vi "TCU Module (Main).vi"(7 "Name of Parent Panel":string="Main.vi", 9 "New Center Coords":T1={"Horizontal"=470, "Vertical"=200}, 10 "Config":variant, 11 "Main UI Message Queue":refnum<queue>) -> ()   [LabVIEW 2018, in "TCU Module.lvlib"]
doc: "This Continuous Measurement sample project is based on the Queued Message Handler template.\n\nThe Event Handling Loop generates messages based on user interface actions.\n\nThe Message Handling Loop processes messages generated by the Event Handling Loop, or by other messages. There are also Acquisition and Logging message handling loop subVIs, and a chart updating loop."
uses:
  TCU Module.lvlib
  support/Message Queue/Message Cluster.ctl
  <vilib>/Utility/miscctls.llb/LVPoint32TypeDef.ctl
  controls/UI Data.ctl
  controls/UI State.ctl
  TCU Module State Cluster.ctl
  TCU Module Config Cluster.ctl
  TCU Module Settings Cluster.ctl
  Measure Instrument/Output Devices.ctl
  Huber TCU/Huber Settings.ctl
  Lauda Integral XT-150 TCU/Lauda Settings.ctl
  Julabo Type 1 TCU/Julabo Type 1 TCU Folder/Julabo FP-50 Settings.ctl
  Huber Unistat 410 TCU/Huber Unistat 410 RS485 Settings.ctl
  Measure Instrument/State Enum.ctl
  TCU Module Display.ctl
  Sequencing/Squence Update Cluster.ctl
  support/Message Queue/Enqueue Message (Single).vi
  support/User Event - Stop/User Event - Stop.lvlib
  support/Support Library.lvlib
  support/Message Queue/Message Queue.lvlib
  Measure Instrument/TCU Module Engine.lvlib
  Measure Instrument/Feed Module Engine.lvlib
  Huber TCU/Huber Ministat 230 TCU.lvlib
  Lauda Integral XT-150 TCU/Lauda TCU.lvlib
  Julabo Type 1 TCU/Julabo Type 1 TCU Folder/Julabo Type FP-50 TCU.lvlib
  Sequencing/Sequencing Library.lvlib
  support/Command Log VIs/Command Logging.lvlib
  Huber Unistat 410 TCU/Huber Unistat 410 TCU.lvlib
panel:
  out "TCU On?":bool
  in  "Settings Button":bool
  out "TCU Image":u16(ring)
  out "ScanCode":i16
  out "Temp Display":dbl
  out "Log File path":path
  out "Status":string
  in  "Exit":bool
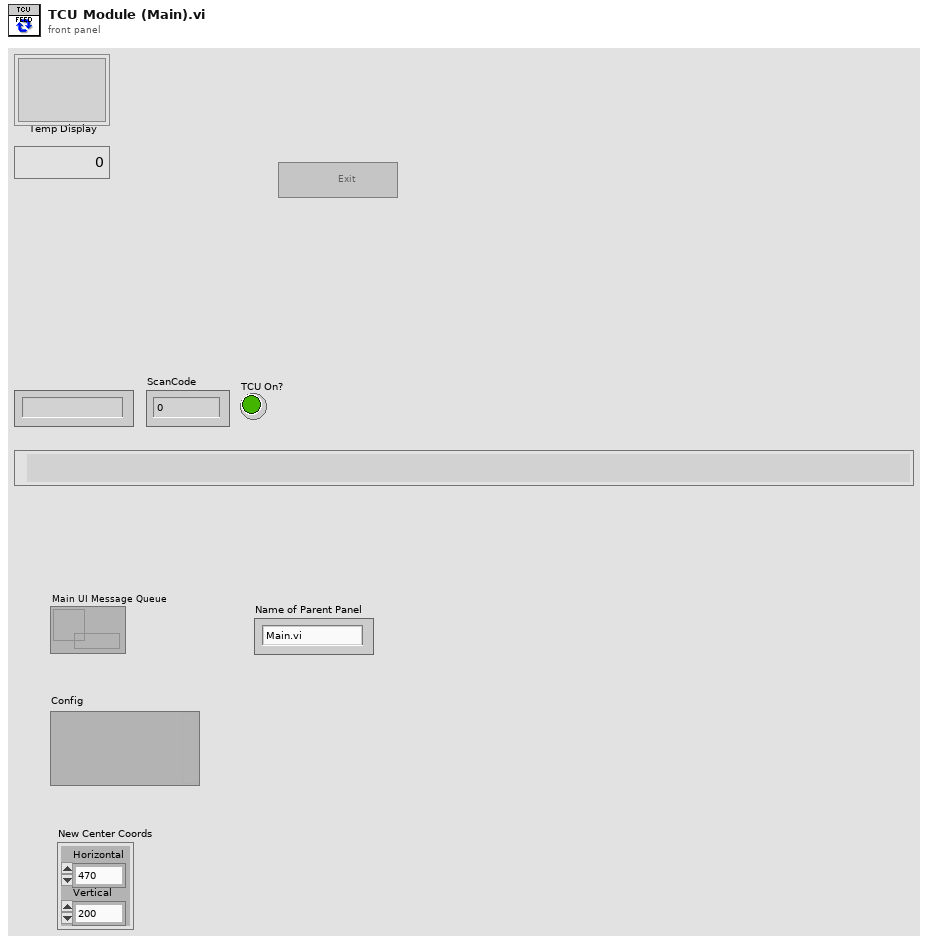
[diagram p1: front panel]
types:
  T1 = typedef "LVPoint32TypeDef.ctl" = cluster{"Horizontal":i32, "Vertical":i32}
  T2 = typedef "TCU Module.lvlib/TCU Module Config Cluster.ctl" = cluster{"GUID":string, "Drop Coords":T1, "Process Name":string, "Queue Name":string, "Settings":T3, "Load Count":i32, "Power Level Changed":bool}
  T3 = typedef "TCU Module.lvlib/TCU Module Settings Cluster.ctl" = cluster{"Cycle Period":dbl, "Setpoint Entry":dbl, "Output Device":T4, "Huber Ministat 230 Settings":T5, "Lauda Settings":T6, "Julabo FP-50 Settings":T7, "Internal Control?":bool, "Huber Unistat 410 Settings":T8}
  T4 = typedef "Output Devices.ctl" = enum16{"Default", "Huber Ministat 230", "Huber Unistat 410", "Lauda XT-150", "Julabo FP-50"}
  T5 = typedef "Huber Ministat 230 TCU.lvlib/Huber Settings.ctl" = cluster{"VISA resource name":refnum<visa-resource-name>, "Simulated?":bool}
  T6 = typedef "Lauda TCU.lvlib/Lauda Settings.ctl" = cluster{"VISA resource name":refnum<visa-resource-name>, "Simulated?":bool, "Pump Power":i32}
  T7 = typedef "Julabo Type FP-50 TCU.lvlib/Julabo FP-50 Settings.ctl" = cluster{"VISA resource name":refnum<visa-resource-name>, "Simulated?":bool, "Pump Power":i32}
  T8 = typedef "Huber Unistat 410 TCU.lvlib/Huber Unistat 410 RS485 Settings.ctl" = cluster{"VISA resource name":refnum<visa-resource-name>, "Address":i8, "Simulated?":bool}
  T9 = typedef "TCU Module.lvlib/TCU Module State Cluster.ctl" = cluster{"TCU Module Config":T2, "State":T10, "Start Time":timestamp, "Current Time":timestamp, "First Iteration":bool, "Data":cluster{"TCU Temp":dbl}, "Process Name":string, "TCU On?":bool, "Power Level Changed":bool}
  T10 = typedef "Feed Module.lvlib/Feed Module Engine.lvlib/State Enum.ctl" = enum16{"Measuring", "Idle", "Paused"}
  T11 = typedef "UI State.ctl" = enum16{"Idle", "Acquiring and Logging", "Waiting for Exit", "Waiting for Exit (Acq Stopped)", "Waiting for Exit (Log Stopped)", "Waiting for Stop", "Waiting for Stop (Acq Stopped)", "Waiting for Stop (Log Stopped)"}
  T12 = typedef "UI Data.ctl" = cluster{"Start Ref":refnum<vi>, "Trigger Ref":refnum<vi>, "Stop Ref":refnum<vi>, "Settings Ref":refnum<vi>, "Status Ref":refnum<vi>, "Exit Ref":refnum<vi>, "Data Ref":refnum<vi>}
  T13 = typedef "TCU Module.lvlib/All Message Queues.ctl" = cluster{"Engine":refnum<queue>, "TCU UI":refnum<queue>, "TCU Engine":refnum<queue>, "TCU Display":refnum<queue>}
  T14 = typedef "TCU Module.lvlib/TCU Module Display.ctl" = cluster{"TCU On?":bool, "Cycle Period":dbl, "Current TCU Temp":dbl}
  T15 = cluster{"Shift":bool, "Ctrl":bool, "Alt":bool, "Cmd":bool, "Opt":bool}
  T16 = typedef "Sequencing Library.lvlib/Squence Update Cluster.ctl" = cluster{"Auto?":bool, "Manual Entry":dbl, "Setpoint":dbl}
  T17 = enum8{"Enabled", "Disabled", "Disabled and Grayed Out"}
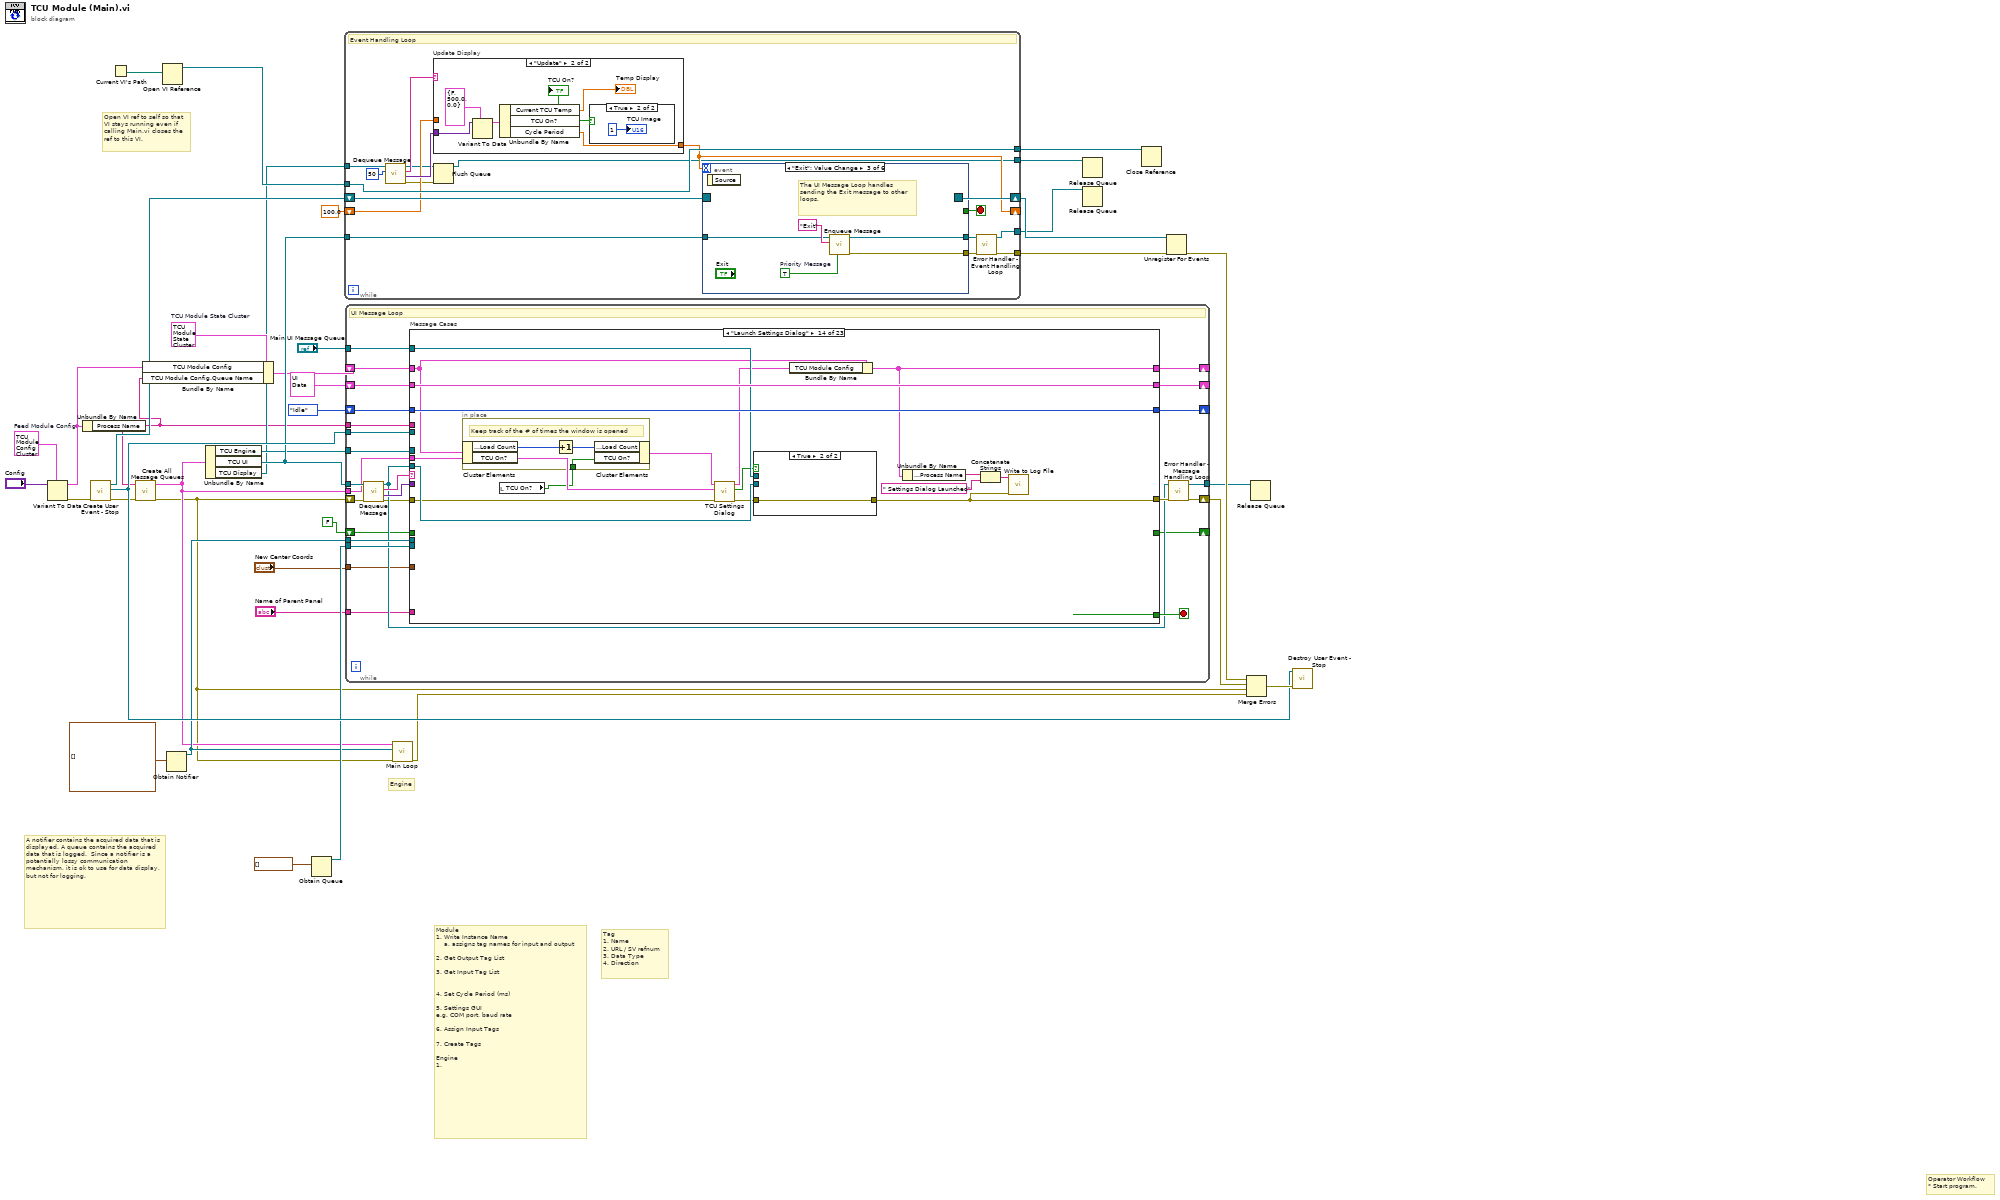
[diagram p0: block diagram]
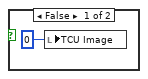
[diagram p3: hidden frame]
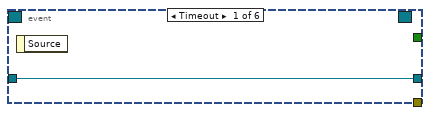
[diagram p4: hidden frame]
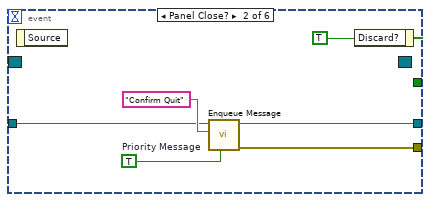
[diagram p5: hidden frame]
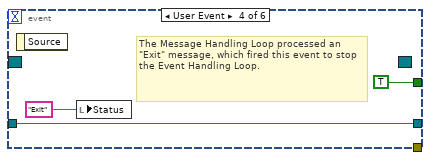
[diagram p6: hidden frame]
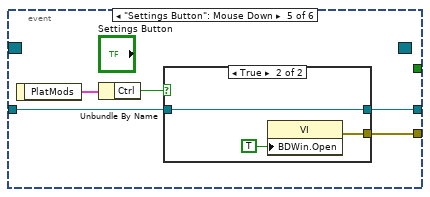
[diagram p7: hidden frame]
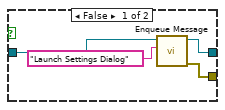
[diagram p8: hidden frame]
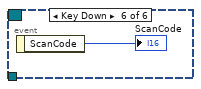
[diagram p9: hidden frame]
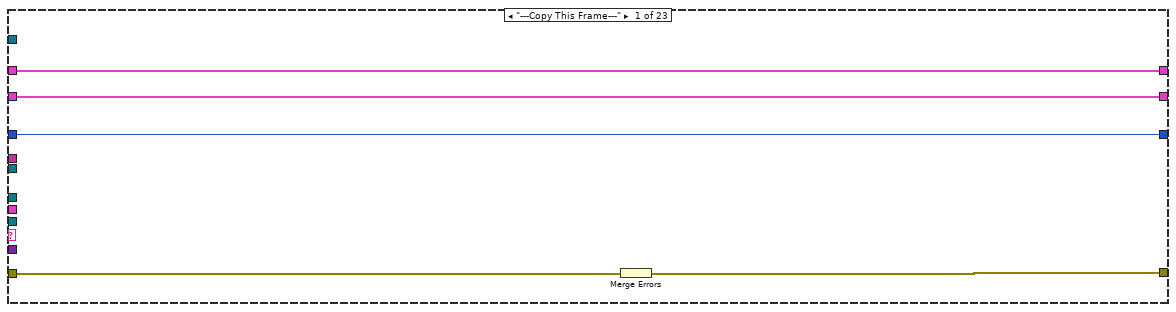
[diagram p10: hidden frame]
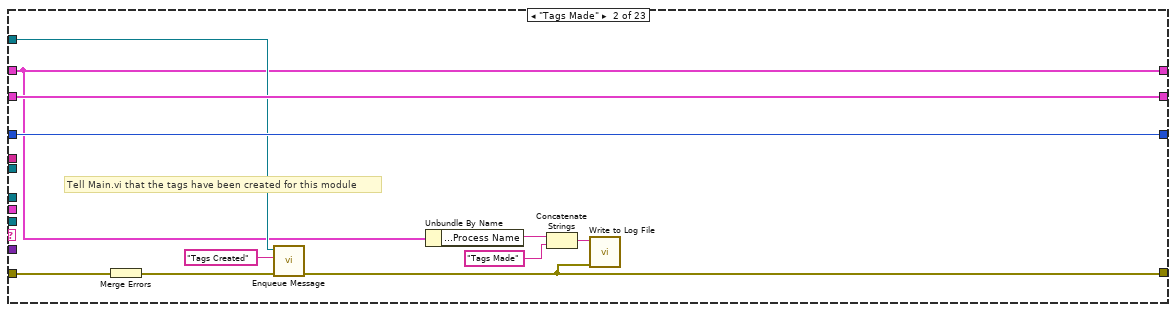
[diagram p11: hidden frame]
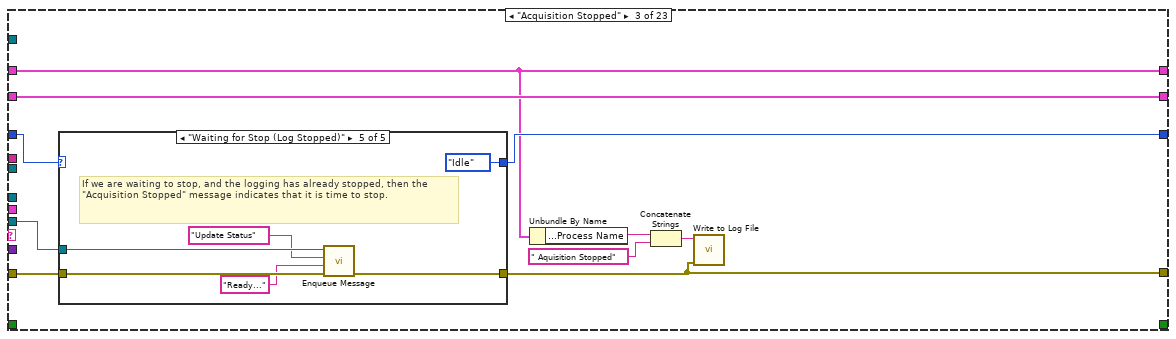
[diagram p12: hidden frame]
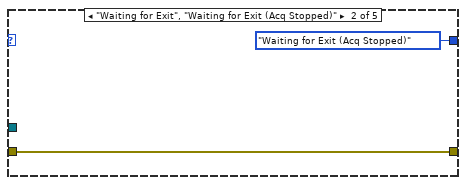
[diagram p14: hidden frame]
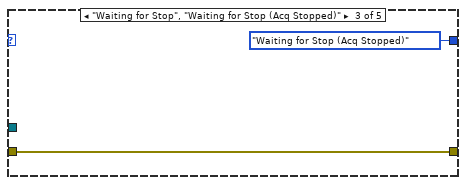
[diagram p15: hidden frame]
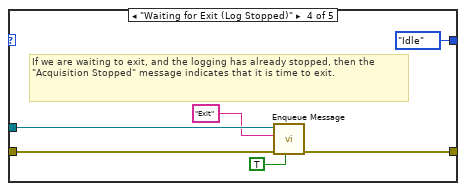
[diagram p16: hidden frame]
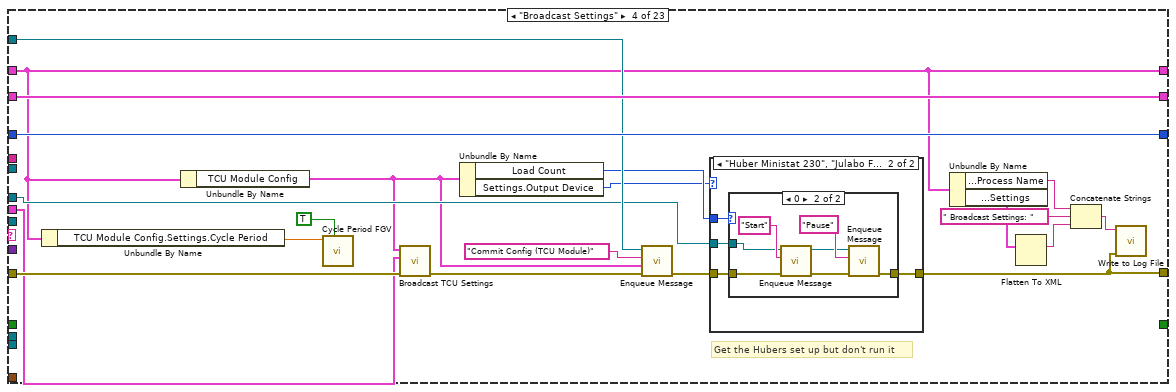
[diagram p17: hidden frame]
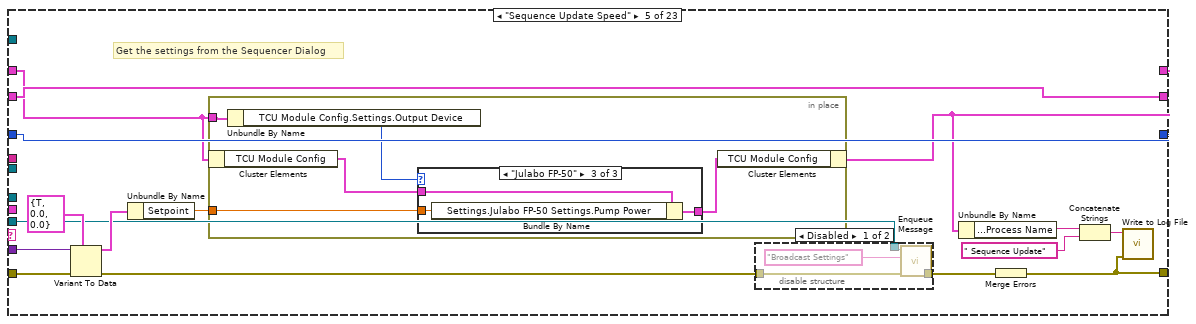
[diagram p20: hidden frame]
diagram:
  w12 = T2 {"GUID"="", "Drop Coords"={"Horizontal"=0, "Vertical"=0}, "Process Name"="", "Queue Name"="", "Settings"={"Cycle Period"=500.0, "Setpoint Entry"=0.0, "Output Device"=enum."Default", "Huber Ministat 230 Settings"={"VISA resource name"="", "Simulated?"=TRUE}, "Lauda Settings"={"VISA resource name"="", "Simulated?"=FALSE, "Pump Power"=2}, "Julabo FP-50 Settings"={"VISA resource name"="", "Simulated?"=FALSE, "Pump Power"=2}, "Internal Control?"=FALSE, "Huber Unistat 410 Settings"={"VISA resource name"="", "Address"=0, "Simulated?"=FALSE}}, "Load Count"=0, "Power Level Changed"=FALSE}  # Feed Module Config
  w15 = T9 {"TCU Module Config"={"GUID"="", "Drop Coords"={"Horizontal"=0, "Vertical"=0}, "Process Name"="", "Queue Name"="", "Settings"={"Cycle Period"=500.0, "Setpoint Entry"=0.0, "Output Device"=enum."Default", "Huber Ministat 230 Settings"={"VISA resource name"="", "Simulated?"=TRUE}, "Lauda Settings"={"VISA resource name"="", "Simulated?"=FALSE, "Pump Power"=2}, "Julabo FP-50 Settings"={"VISA resource name"="", "Simulated?"=FALSE, "Pump Power"=2}, "Internal Control?"=FALSE, "Huber Unistat 410 Settings"={"VISA resource name"="", "Address"=0, "Simulated?"=FALSE}}, "Load Count"=0, "Power Level Changed"=FALSE}, "State"=enum."Idle", "Start Time"=timestamp(0 s since 1904-01-01), "Current Time"=timestamp(0 s since 1904-01-01), "First Iteration"=FALSE, "Data"={"TCU Temp"=0.0}, "Process Name"="", "TCU On?"=FALSE, "Power Level Changed"=FALSE}  # TCU Module State Cluster
  # "Open VI ref to self so that\nVI stays running even if\ncalling Main.vi closes the\nref to this VI."
  # "Engine"
  # "Operator Workflow\n* Start program."
  # "Module \n1. Write Instance Name\n    a. assigns tag names for input and output\n\n2. Get Output Tag List\n\n3. Get Input Tag List\n\n\n4. Set Cycle Period (ms)\n\n5. Settings GUI\ne.g. COM port, baud rate\n\n6. Assign Input Tags\n\n7. Create Tags\n\nEngine\n1."
  # "Tag\n1. Name\n2. URL / SV refnum\n3. Data Type\n4. Direction"
  # "A notifier contains the acquired data that is displayed. A queue contains the acquired data that is logged.  Since a notifier is a potentially lossy communication mechanism, it is ok to use for data display, but not for logging."
  n1 = Variant To Data(type=w12, Variant="Config") -> (data=w17:T2, error out=w18:errorcluster)  [unwired: 1 in]
  n2 = Unbundle By Name(w17) -> ("Process Name"=w5:string)
  n3 = call "Create User Event - Stop.vi"("error in (no error)"=w18) -> ("error out"=w11:errorcluster, "User Event - Stop"=w34:refnum<user-event>, "Stop Event Registration Refnum"=w35:refnum<event-registration>)  [unwired: 8 in]
  n4 = Current VI's Path() -> (path=w20:path)
  n5 = call "Create All Message Queues.vi"("error in (no error)"=w11, "Process Name"=w5) -> ("error out"=w9:errorcluster, "Message Queues"=w10:T13)  [unwired: 8 in]
  n6 = Bundle By Name(cluster=w15, "TCU Module Config"=w17, "TCU Module Config.Queue Name"=w5) -> (w19:T9)
  n7 = Open VI Reference(vi path=w20) -> (vi reference=w21:refnum<vi>)  [unwired: 5 in, 1 out]
  n8 = Obtain Notifier(notification data type=waveform(dbl)[] []) -> (notifier out=w23:refnum<notifier>)  [unwired: 3 in, 2 out]
  n9 = Unbundle By Name(w10) -> ("TCU Engine"=w26:refnum<queue>, "TCU UI"=w30:refnum<queue>, "TCU Display"=w14:refnum<queue>)
  n10 = Obtain Queue(element data type=waveform(dbl)[] []) -> (queue out=w25:refnum<queue>)  [unwired: 4 in, 2 out]
  n11 = while {
    tunnel: w30 -> [w50]
    tunnel: [w52] -> w37
    shift-right: [w51] -> w32
    shift-left: w35 -> [w56]
    tunnel: [w49] -> w22
    tunnel: w21 -> [w49]
    tunnel: w14 -> [w48]
    shift-right: [w45] -> _
    shift-left: 100.0 ("Cycle Period") -> [w44]
    tunnel: [w40] -> w2
    tunnel: [w39] -> w3
    stop <- w55 stop-if-true
    # "Event Handling Loop"
    n12 = call "Dequeue Message.vi"("timeout in ms (-1)"=50, "Message Queue"=w48) -> ("error out"=w41:errorcluster, "Message Data"=w46:variant, "Message"=w47:string, "dup Message Queue"=w42:refnum<queue>)  [unwired: 6 in]
    n13 = case "Update Display" shown="\"Update\"" w47 {
      tunnel: w46 -> [_ w63]
      tunnel: [w57 w59] -> w45
      tunnel: w44 -> [w57 _]
      frame "False", Default {
      }
      frame "Update" {
        n14 = Variant To Data(type=T14 {"TCU On?"=FALSE, "Cycle Period"=500.0, "Current TCU Temp"=0.0} ("FM Display"), Variant=w63) -> (data=w62:T14)  [unwired: 1 in, 1 out]
        n15 = Unbundle By Name(w62) -> ("Current TCU Temp"=→"Temp Display":dbl, "TCU On?"=w60:bool, "Cycle Period"=w59:dbl)
        "TCU On?" <- w60
        n16 = case shown="True" w60 {
          frame False {
            n17 = local write "TCU Image"(u16 0 ("Ring")) -> ()
          }
          frame True {
            "TCU Image" <- u16 1 ("Ring")
          }
        }
      }
    }
    n18 = Flush Queue(queue=w42, error in (no error)=w41) -> (queue out=w39:refnum<queue>)  [unwired: 2 out]
    n19 = event shown="[2] \"Exit\": Value Change" {
      selector: w56 -> [_ _ _ _ _ _]
      dyn-events: [_ _ _ _ _ _] -> w51
      timeout: w45 -> [_ _ _ _ _ _]
      tunnel: [_ _ _ TRUE ("Discard?") _ _] -> w55
      tunnel: w50 -> [w66 w69 w74 w78 w83 _]
      tunnel: [_ w67 w77 _ w85 _] -> w53
      tunnel: [w66 w68 w73 w78 w84 _] -> w54
      event Timeout {
        n20 = event-data() -> ()  [unwired: 1 in, 1 out]
      }
      event Panel Close? {
        w70 = TRUE  # Priority Message
        n21 = event-data() -> ()  [unwired: 1 in, 1 out]
        n22 = call-poly "Enqueue Message.vi"("Priority Message? (F)"=w70, "Message"="Confirm Quit", "Message Queue"=w69) -> ("error out"=w67:errorcluster, "dup Message Queue"=w68:refnum<queue>)  [unwired: 7 in]
        n23 = event-data("Discard?"=TRUE) -> ()  [unwired: 1 in, 1 out]
      }
      event "Exit": Value Change {
        w75 = TRUE  # Priority Message
        # "The UI Message Loop handles sending the Exit message to other loops."
        n24 = event-data() -> ()  [unwired: 1 in, 1 out]
        n25 = call-poly "Enqueue Message.vi"("Priority Message? (F)"=w75, "Message"="Exit", "Message Queue"=w74) -> ("error out"=w77:errorcluster, "dup Message Queue"=w73:refnum<queue>)  [unwired: 7 in]
      }
      event User Event {
        # "The Message Handling Loop processed an \"Exit\" message, which fired this event to stop the Event Handling Loop."
        n26 = event-data() -> ()  [unwired: 1 in, 1 out]
        n27 = local write "Status"("Exit" ("Exit String")) -> ()
      }
      event "Settings Button": Mouse Down {
        n28 = event-data() -> ("PlatMods"=w82:T15)  [unwired: 1 in]
        n29 = Unbundle By Name(w82) -> ("Ctrl"=w81:bool)
        n30 = case shown="True" w81 {
          tunnel: [w89 w90] -> w85
          tunnel: [w88 w91] -> w84
          tunnel: w83 -> [w87 w91]
          frame False {
            n31 = call-poly "Enqueue Message.vi"("Message"="Launch Settings Dialog", "Message Queue"=w87) -> ("error out"=w89:errorcluster, "dup Message Queue"=w88:refnum<queue>)  [unwired: 8 in]
          }
          frame True {
            n32 = property class="VI"("BDWin.Open"=TRUE ("Block Diagram Window:Open")) -> (error out=w90:errorcluster)  [unwired: 2 in, 1 out]
          }
        }
      }
      event Key Down {
        n33 = event-data() -> ("ScanCode"=→"ScanCode":i16)  [unwired: 1 in]
      }
    }
    n34 = call "Error Handler - Event Handling Loop.vi"("error in (no error)"=w53, "Message Queue"=w54) -> ("dup error in"=w52:errorcluster, "dup Message Queue"=w40:refnum<queue>)  [unwired: 8 in]
  }
  n35 = while {
    tunnel: w30 -> [w115]
    tunnel: w34 -> [w119]
    shift-right: [w109] -> w38
    shift-left: w9 -> [w118]
    shift-right: [w101] -> _
    shift-left: w19 -> [w103]
    shift-right: [w113] -> _
    shift-left: T12 {"Start Ref"=refnum, "Trigger Ref"=refnum, "Stop Ref"=refnum, "Settings Ref"=refnum, "Status Ref"=refnum, "Exit Ref"=refnum, "Data Ref"=refnum} ("Measurement UI Controls") -> [w114]
    tunnel: w23 -> [w112]
    tunnel: w25 -> [w111]
    shift-right: [w106] -> _
    shift-left: UI_State."Idle" ("UI State") -> [w107]
    tunnel: w26 -> [w105]
    tunnel: "Main UI Message Queue" -> [w102]
    tunnel: w10 -> [w100]
    tunnel: w5 -> [w99]
    tunnel: "New Center Coords" -> [w98]
    tunnel: "Name of Parent Panel" -> [w97]
    shift-right: [w96] -> _
    shift-left: FALSE -> [w95]
    tunnel: [w94] -> w1
    stop <- w120 stop-if-true
    # "UI Message Loop"
    n36 = call "Dequeue Message.vi"("error in (no error)"=w118, "Message Queue"=w115) -> ("error out"=w104:errorcluster, "Message Data"=w116:variant, "Message"=w117:string, "dup Message Queue"=w108:refnum<queue>)  [unwired: 6 in]
    n37 = case "Message Cases" shown="\"Launch Settings Dialog\"" w117 {
      selector: w117 -> [_ _ _ _ _ _ _ _ _ _ _ _ _ _ _ _ _ _ _ _ _ _ w620]
      tunnel: w108 -> [_ _ w142 _ w207 w239 w258 _ w325 w339 w364 _ w402 w422 w443 _ w489 w520 _ _ w573 _ _]
      tunnel: w104 -> [w125 w136 w143 w181 w206 w238 w257 w293 w306 w343 w368 w387 w397 w420 w444 w469 w487 w519 w539 w553 w571 w612 _]
      tunnel: [w124 w126 w139 w168 w201 w233 w255 w294 w300 w330 w346 w387 w389 w413 w439 w473 w478 w505 w547 w555 w576 w613 w619] -> w110
      tunnel: [_ _ _ _ _ _ _ _ _ _ TRUE _ _ _ _ _ _ _ _ _ _ _ _] -> w120
      tunnel: w116 -> [_ _ _ _ w205 w237 _ w296 _ w342 w350 _ _ _ _ w466 _ _ _ _ _ w611 _]
      tunnel: w119 -> [_ _ _ _ _ _ _ _ _ _ w367 _ _ _ _ _ _ _ _ _ _ _ _]
      tunnel: w103 -> [w121 w127 w138 w167 w200 w232 w254 w291 w304 w329 w345 w378 w388 w410 w438 w471 w483 w515 w540 w554 w581 w602 w625]
      tunnel: w114 -> [w123 w135 w146 w185 w209 w241 w260 w298 w322 w344 w365 w386 w398 w425 w447 w476 w484 w516 w546 w564 w597 w608 w630]
      tunnel: [w123 w135 w146 w185 w209 w241 w260 w298 w322 w344 w365 w385 w398 w425 w447 w476 w484 w516 w546 w564 w597 w608 w630] -> w113
      tunnel: w112 -> [_ _ _ _ _ _ _ _ _ _ w363 _ _ _ _ _ _ _ _ _ _ _ _]
      tunnel: w111 -> [_ _ _ _ _ _ _ _ _ _ w359 _ _ _ _ _ _ _ _ _ _ _ _]
      tunnel: w107 -> [w122 w134 w145 w184 w208 w240 w259 w292 w311 w334 _ _ _ w424 w446 w472 _ _ _ _ w586 w603 w629]
      tunnel: [w122 w134 w144 w184 w208 w240 w256 w292 w312 w334 UI_State."Idle" ("UI State") UI_State."Idle" ("UI State") UI_State."Idle" ("UI State") w424 w445 w472 UI_State."Acquiring and Logging" ("UI State") UI_State."Acquiring and Logging" ("UI State") UI_State."Acquiring and Logging" ("UI State") UI_State."Acquiring and Logging" ("UI State") w587 w603 w629] -> w106
      tunnel: w105 -> [_ _ _ w174 _ _ _ _ w310 _ w357 _ _ _ _ _ _ _ w544 w562 w585 _ _]
      tunnel: w102 -> [_ w132 _ w180 _ _ _ _ _ _ w351 _ _ w423 _ _ _ _ _ _ _ _ _]
      tunnel: [w121 w127 w138 w167 w199 w231 w254 w291 w299 w329 w345 w378 w388 w412 w438 w471 w477 w504 w540 w554 w575 w602 w625] -> w101
      tunnel: w100 -> [_ _ _ w177 _ _ _ _ _ _ _ _ _ w417 _ _ _ _ _ _ _ _ _]
      tunnel: w99 -> [_ _ _ _ _ _ _ _ _ _ _ _ w393 _ _ _ _ _ _ _ _ _ _]
      tunnel: w98 -> [_ _ _ _ _ _ _ _ _ _ _ _ w395 _ _ _ _ _ _ _ _ _ _]
      tunnel: w97 -> [_ _ _ _ _ _ _ _ _ _ _ _ w394 _ _ _ _ _ _ _ _ _ _]
      tunnel: w95 -> [_ _ _ _ _ _ _ _ _ _ _ _ _ _ _ _ _ w510 _ _ _ _ _]
      tunnel: [_ _ _ _ _ _ _ _ _ _ _ _ _ _ _ _ _ w509 _ _ _ _ _] -> w96
      frame "---Copy This Frame---" {
        # "Duplicate this frame when creating new messages.  Change this comment in the duplicated frame to describe this message."
        n38 = Merge Errors(w125) -> (w124:errorcluster)
      }
      frame "Tags Made" {
        # "Tell Main.vi that the tags have been created for this module"
        # "Duplicate this frame when creating new messages.  Change this comment in the duplicated frame to describe this message."
        n39 = Merge Errors(w136) -> (w131:errorcluster)
        n40 = call-poly "Enqueue Message.vi"("error in (no error)"=w131, "Message"="Tags Created", "Message Queue"=w132) -> ("error out"=w126:errorcluster)  [unwired: 7 in, 1 out]
        n41 = Unbundle By Name(w127) -> ("TCU Module Config.Process Name"=w130:string)
        n42 = Concatenate Strings(w130, "Tags Made" ("text")) -> (w128:string)
        n43 = call "Write to Log File.vi"("error in"=w126, "text"=w128) -> ()  [unwired: 9 in, 1 out]
      }
      frame "Acquisition Stopped" {
        # "Logic for determining what action to take when the acquisition has stopped."
        n44 = case shown="\"Waiting for Stop (Log Stopped)\"" w145 {
          selector: w145 -> [w148 _ _ _ _]
          tunnel: [w148 UI_State."Waiting for Exit (Acq Stopped)" ("UI State") UI_State."Waiting for Stop (Acq Stopped)" ("UI State") UI_State."Idle" ("UI State") UI_State."Idle" ("UI State")] -> w144
          tunnel: w143 -> [w147 w149 w151 w157 w163]
          tunnel: [w147 w149 w151 w156 w162] -> w139
          tunnel: w142 -> [_ _ _ w155 w161]
          frame Default {
          }
          frame "Waiting for Exit", "Waiting for Exit (Acq Stopped)" {
          }
          frame "Waiting for Stop", "Waiting for Stop (Acq Stopped)" {
          }
          frame "Waiting for Exit (Log Stopped)" {
            # "If we are waiting to exit, and the logging has already stopped, then the \"Acquisition Stopped\" message indicates that it is time to exit."
            n45 = call-poly "Enqueue Message.vi"("Priority Message? (F)"=TRUE, "error in (no error)"=w157, "Message"="Exit", "Message Queue"=w155) -> ("error out"=w156:errorcluster)  [unwired: 6 in, 1 out]
          }
          frame "Waiting for Stop (Log Stopped)" {
            # "If we are waiting to stop, and the logging has already stopped, then the \"Acquisition Stopped\" message indicates that it is time to stop."
            n46 = call-poly "Enqueue Message.vi"("error in (no error)"=w163, "Message Data"="Ready..." ("Message"), "Message"="Update Status", "Message Queue"=w161) -> ("error out"=w162:errorcluster)  [unwired: 6 in, 1 out]
          }
        }
        n47 = Unbundle By Name(w138) -> ("TCU Module Config.Process Name"=w141:string)
        n48 = Concatenate Strings(w141, " Aquisition Stopped" ("text")) -> (w140:string)
        n49 = call "Write to Log File.vi"("error in"=w139, "text"=w140) -> ()  [unwired: 9 in, 1 out]
      }
      frame "Broadcast Settings" {
        # "Get the Hubers set up but don't run it"
        # "Send the 'Update Settings' message to the Logging and Acquisition message loops."
        n50 = Unbundle By Name(w167) -> ("TCU Module Config.Settings.Cycle Period"=w182:dbl)
        n51 = Unbundle By Name(w167) -> ("TCU Module Config"=w172:T2)
        n52 = call "Cycle Period FGV.vi"("Write"=TRUE, "Cycle Period In (ms)"=w182) -> ()  [unwired: 8 in, 2 out]
        n53 = call "Broadcast TCU Settings.vi"("error in (no error)"=w181, "Message Queues"=w177, "Pump Module Config"=w172) -> ("error out"=w179:errorcluster)  [unwired: 8 in]
        n54 = Unbundle By Name(w172) -> ("Load Count"=w176:i32, "Settings.Output Device"=w173:T4)
        n55 = call-poly "Enqueue Message.vi"("error in (no error)"=w179, "Message Data"=w172, "Message"="Commit Config (TCU Module)", "Message Queue"=w180) -> ("error out"=w175:errorcluster)  [unwired: 6 in, 1 out]
        n56 = case shown="\"Huber Ministat 230\", \"Julabo FP-50\"" w173 {
          tunnel: w175 -> [w186 w190]
          tunnel: w174 -> [_ w189]
          tunnel: [w186 w188] -> w168
          tunnel: w176 -> [_ w187]
          frame "Default", Default {
          }
          frame "Huber Ministat 230", "Julabo FP-50" {
            n57 = case shown="0" w187 {
              tunnel: w190 -> [w191 w195]
              tunnel: w189 -> [_ w194]
              tunnel: [w191 w198] -> w188
              frame Default {
              }
              frame 0 {
                n58 = call-poly "Enqueue Message.vi"("error in (no error)"=w195, "Message"="Start", "Message Queue"=w194) -> ("error out"=w192:errorcluster, "dup Message Queue"=w193:refnum<queue>)  [unwired: 7 in]
                n59 = call-poly "Enqueue Message.vi"("error in (no error)"=w192, "Message"="Pause", "Message Queue"=w193) -> ("error out"=w198:errorcluster)  [unwired: 7 in, 1 out]
              }
            }
          }
        }
        n60 = Unbundle By Name(w167) -> ("TCU Module Config.Process Name"=w171:string, "TCU Module Config.Settings"=w166:T3)
        n61 = Flatten To XML(anything=w166) -> (xml string=w165:string)
        n62 = Concatenate Strings(w171, " Broadcast Settings: " ("text"), w165) -> (w170:string)
        n63 = call "Write to Log File.vi"("error in"=w168, "text"=w170) -> ()  [unwired: 9 in, 1 out]
      }
      frame "Sequence Update Speed" {
        # "Get the settings from the Sequencer Dialog"
        # "Send the 'Update Settings' message to the Logging and Acquisition message loops."
        n64 = Variant To Data(error in=w206, type=T16 {"Auto?"=TRUE, "Manual Entry"=0.0, "Setpoint"=0.0} ("Cluster"), Variant=w205) -> (data=w213:T16, error out=w210:errorcluster)
        n65 = Unbundle By Name(w213) -> ("Setpoint"=w212:dbl)
        n66 = in-place {
          in-place-border: w212 -> [w223]
          in-place-border: w200 -> [w222]
          n67 = in-place-cluster #1(w200) -> ("TCU Module Config"=w220:T2)
          n68 = Unbundle By Name(w222) -> ("TCU Module Config.Settings.Output Device"=w221:T4)
          n69 = case shown="\"Julabo FP-50\"" w221 {
            tunnel: w220 -> [w224 w227 w230]
            tunnel: w223 -> [_ w226 w229]
            tunnel: [w224 w225 w228] -> w219
            frame "Default", Default {
            }
            frame "Lauda XT-150" {
              n70 = Bundle By Name(cluster=w227, "Settings.Lauda Settings.Pump Power"=w226) -> (w225:T2)
            }
            frame "Julabo FP-50" {
              n71 = Bundle By Name(cluster=w230, "Settings.Julabo FP-50 Settings.Pump Power"=w229) -> (w228:T2)
            }
          }
          n72 = in-place-cluster #1("TCU Module Config"=w219) -> (w199:T9)
        }
        n73 = disable-structure shown="Disabled" {
          disable-tunnel: [w218 _] -> w211
          disable-tunnel: w210 -> [w216 _]
          disable-tunnel: w207 -> [w215 _]
          frame Disabled {
            n74 = call-poly "Enqueue Message.vi"("error in (no error)"=w216, "Message"="Broadcast Settings", "Message Queue"=w215) -> ("error out"=w218:errorcluster)  [unwired: 7 in, 1 out]
          }
          frame Enabled {
          }
        }
        n75 = Unbundle By Name(w199) -> ("TCU Module Config.Process Name"=w204:string)
        n76 = Merge Errors(w211) -> (w201:errorcluster)
        n77 = Concatenate Strings(w204, " Sequence Update" ("text")) -> (w203:string)
        n78 = call "Write to Log File.vi"("error in"=w201, "text"=w203) -> ()  [unwired: 9 in, 1 out]
      }
      frame "Sequence Update Temperature" {
        # "Get the settings from the Sequencer Dialog"
        # "Send the 'Update Settings' message to the Logging and Acquisition message loops."
        n79 = Variant To Data(error in=w238, type=T16 {"Auto?"=TRUE, "Manual Entry"=0.0, "Setpoint"=0.0} ("Cluster"), Variant=w237) -> (data=w245:T16, error out=w242:errorcluster)
        n80 = Unbundle By Name(w245) -> ("Setpoint"=w244:dbl)
        n81 = in-place {
          in-place-border: w244 -> [w253]
          n82 = in-place-cluster #2(w232) -> ("TCU Module Config"=w251:T2)
          n83 = Bundle By Name(cluster=w251, "Settings.Setpoint Entry"=w253) -> (w252:T2)
          n84 = in-place-cluster #2("TCU Module Config"=w252) -> (w231:T9)
        }
        n85 = disable-structure shown="Disabled" {
          disable-tunnel: [w250 _] -> w243
          disable-tunnel: w242 -> [w248 _]
          disable-tunnel: w239 -> [w247 _]
          frame Disabled {
            n86 = call-poly "Enqueue Message.vi"("error in (no error)"=w248, "Message"="Broadcast Settings", "Message Queue"=w247) -> ("error out"=w250:errorcluster)  [unwired: 7 in, 1 out]
          }
          frame Enabled {
          }
        }
        n87 = Unbundle By Name(w231) -> ("TCU Module Config.Process Name"=w236:string)
        n88 = Merge Errors(w243) -> (w233:errorcluster)
        n89 = Concatenate Strings(w236, " Sequence Update" ("text")) -> (w235:string)
        n90 = call "Write to Log File.vi"("error in"=w233, "text"=w235) -> ()  [unwired: 9 in, 1 out]
      }
      frame "Confirm Quit" {
        # "Confirm Quit - Message that can confirm whether or not the user wants to exit the application."
        n91 = case shown="\"Acquiring and Logging\"" w259 {
          tunnel: w258 -> [w269 w276]
          tunnel: w257 -> [w268 w274]
          tunnel: [w262 w273] -> w255
          tunnel: [UI_State."Idle" ("UI State") w272] -> w256
          tunnel: w254 -> [w261 w271]
          frame Default {
            # "If 'Confirm Quit' comes in while the system is idle, there is no need for a confirmation message."
            n92 = call-poly "Enqueue Message.vi"("Priority Message? (F)"=TRUE, "error in (no error)"=w268, "Message"="Exit", "Message Queue"=w269) -> ("error out"=w262:errorcluster)  [unwired: 6 in, 1 out]
            n93 = Unbundle By Name(w261) -> ("TCU Module Config.Process Name"=w265:string)
            n94 = Concatenate Strings(w265, " Quit" ("text")) -> (w264:string)
            n95 = call "Write to Log File.vi"("error in"=w262, "text"=w264) -> ()  [unwired: 9 in, 1 out]
          }
          frame "Acquiring and Logging" {
            n96 = Two Button Dialog(message="Are you sure you want to quit while the acquisition is running?" ("Confirm Quit Message"), 1:"No" ("No"), 2:"Yes" ("Yes")) -> (T button?=w275:bool)
            n97 = case shown="True" w275 {
              tunnel: w276 -> [_ w290]
              tunnel: w274 -> [w280 w289]
              tunnel: [w280 w283] -> w273
              tunnel: [UI_State."Acquiring and Logging" ("UI State") UI_State."Waiting for Exit" ("UI State")] -> w272
              tunnel: w271 -> [_ w282]
              frame False {
                # "User did not want to quit."
              }
              frame True {
                n98 = call-poly "Enqueue Message.vi"("error in (no error)"=w289, "Message"="Stop", "Message Queue"=w290) -> ("error out"=w283:errorcluster)  [unwired: 7 in, 1 out]
                n99 = Unbundle By Name(w282) -> ("TCU Module Config.Process Name"=w286:string)
                n100 = Concatenate Strings(w286, " Quit" ("text")) -> (w285:string)
                n101 = call "Write to Log File.vi"("error in"=w283, "text"=w285) -> ()  [unwired: 9 in, 1 out]
              }
            }
          }
        }
      }
      frame "Display Log File Path" {
        n102 = Variant To Data(error in=w293, type=path "", Variant=w296) -> (data=→"Log File path":path, error out=w294:errorcluster)
      }
      frame "E-Stop" {
        # "Pause the TCU when E-Stop is pressed"
        # "Message Acquisition and Logging loops to stop"
        # "Enable: Start, Exit, Settings\nDisable: Stop"
        # "Stop the pumps."
        n103 = Unbundle By Name(w322) -> ("Trigger Ref"=w313:refnum<vi>, "Stop Ref"=w314:refnum<vi>, "Start Ref"=w317:refnum<vi>, "Exit Ref"=w316:refnum<vi>, "Settings Ref"=w315:refnum<vi>)
        n104 = call-poly "Enqueue Message.vi"("error in (no error)"=w306, "Message Data"="Ready..." ("Ready..."), "Message"="Update Status", "Message Queue"=w325) -> ("error out"=w308:errorcluster)  [unwired: 6 in, 1 out]
        n105 = Build Array(w317, w316, w315) -> (w320:refnum<vi>[])
        n106 = Build Array(w313, w314) -> (w319:refnum<vi>[])
        n107 = call-poly "Enqueue Message.vi"("error in (no error)"=w308, "Message"="Pause", "Message Queue"=w310) -> ("error out"=w307:errorcluster)  [unwired: 7 in, 1 out]
        n108 = call "Set Enable State on Multiple Controls.vi"("Enable?"=FALSE, "Controls"=w319) -> ()  [unwired: 10 in]
        n109 = call "Set Enable State on Multiple Controls.vi"("Enable?"=TRUE, "Controls"=w320) -> ()  [unwired: 10 in]
        n110 = case shown="Default" w311 {
          selector: w311 -> [_ w327]
          tunnel: [UI_State."Waiting for Stop" ("UI State") w327] -> w312
          frame Default {
          }
          frame "Waiting for Exit" {
          }
        }
        n111 = Bundle By Name(cluster=w304, "State"=State_Enum."Idle") -> (w299:T9)
        n112 = Merge Errors(w307) -> (w300:errorcluster)
        n113 = Unbundle By Name(w299) -> ("TCU Module Config.Process Name"=w303:string)
        n114 = Concatenate Strings(w303, " E-STOP" ("text")) -> (w302:string)
        n115 = call "Write to Log File.vi"("error in"=w300, "text"=w302) -> ()  [unwired: 9 in, 1 out]
      }
      frame "Error" {
        # "Error - Check the error message data and respond accordingly. This message is sent by the \"Error Handler\" VIs at the end of each loop in this application."
        n116 = Variant To Data(error in=w343, type=errorcluster {"status"=FALSE, "code"=0, "source"=""} ("error out"), Variant=w342) -> (data=w340:errorcluster, error out=w336:errorcluster)
        n117 = call <vilib>:"General Error Handler.vi"("error in (no error)"=w340) -> ("message"=w328:string)  [unwired: 10 in, 4 out]
        n118 = call-poly "Enqueue Message.vi"("Priority Message? (F)"=TRUE, "Message"="Exit", "Message Queue"=w339) -> ("error out"=w335:errorcluster)  [unwired: 7 in, 1 out]
        n119 = Merge Errors(w335, w336) -> (w330:errorcluster)
        n120 = Unbundle By Name(w329) -> ("TCU Module Config.Process Name"=w333:string)
        n121 = Concatenate Strings(w333, " Error: " ("text"), w328) -> (w332:string)
        n122 = call "Write to Log File.vi"("error in"=w330, "text"=w332) -> ()  [unwired: 9 in, 1 out]
      }
      frame "Exit" {
        w354 = TRUE  # Delete Module?
        # "Don't check the error outs. The acquisition and logging queues may have already been released."
        # "Close references owned by the Main VI."
        # "Stop the VI"
        # "Exit - Fire the User Event to stop the Event Handling Loop.  Also send Exit messages to the Acquisition and Logging loops."
        n123 = Release Queue(queue=w364, error in (no error)=w368) -> (error out=w362:errorcluster)  [unwired: 1 in, 2 out]
        n124 = call "Fire User Event - Stop.vi"("User Event - Stop"=w367) -> ("error out"=w366:errorcluster)  [unwired: 10 in]
        n125 = Release Notifier(notifier=w363, error in (no error)=w362) -> (error out=w361:errorcluster)  [unwired: 1 in, 2 out]
        n126 = Build Array(w357) -> (w356:refnum<queue>[])
        n127 = Release Queue(queue=w359, error in (no error)=w361) -> (error out=w360:errorcluster)  [unwired: 1 in, 2 out]
        n128 = for {
          tunnel: w356 -> [w375] mode=indexing
          n129 = call-poly "Enqueue Message.vi"("Message"="Stop", "Message Queue"=w375) -> ("dup Message Queue"=w376:refnum<queue>)  [unwired: 8 in, 1 out]
          n130 = call-poly "Enqueue Message.vi"("Message"="Exit", "Message Queue"=w376) -> ()  [unwired: 8 in, 2 out]
        }
        n131 = Variant To Data(type=w354, Variant=w350) -> (data=w353:bool, error out=w355:errorcluster)  [unwired: 1 in]
        n132 = Select(t=w354, s=w355, f=w353) -> (s? t:f=w352:bool)
        n133 = case "Don't enqueue Delete Module if opening campaign because it\nwill already have been deleted and new config loaded and we create\na race condition." shown="True" w352 {
          tunnel: w351 -> [_ w372]
          tunnel: w345 -> [_ w371]
          frame False {
          }
          frame True {
            n134 = Unbundle By Name(w371) -> ("TCU Module Config.GUID"=w370:string)
            n135 = call-poly "Enqueue Message.vi"("Message Data"=w370, "Message"="Delete Module", "Message Queue"=w372) -> ()  [unwired: 7 in, 2 out]
          }
        }
        n136 = Merge Errors(w366, w360) -> (w346:errorcluster)
        n137 = Unbundle By Name(w345) -> ("TCU Module Config.Process Name"=w349:string)
        n138 = Concatenate Strings(w349, " Exit" ("text")) -> (w348:string)
        n139 = call "Write to Log File.vi"("error in"=w346, "text"=w348) -> ()  [unwired: 9 in, 1 out]
      }
      frame "Init UI Refs" {
        # "Enable: Start, Exit, Settings\nDisable: Stop"
        # "Init UI Refs - Store control references for UI controls.  Also enable/disable controls appropriately."
        n140 = property class="VI"("Front Panel.Closeable"=TRUE ("Front Panel Window:Closeable")) -> ()  [unwired: 2 in, 2 out]
        n141 = control-ref of="Status"() -> (w383:refnum<vi>)
        n142 = control-ref of="Exit"() -> (w380:refnum<vi>)
        n143 = Bundle By Name(cluster=w386, "Status Ref"=w383, "Exit Ref"=w380) -> (w385:T12)
        n144 = Build Array(w380) -> (w382:refnum<vi>[])
        n145 = call "Set Enable State on Multiple Controls.vi"("Enable?"=TRUE, "Controls"=w382) -> ()  [unwired: 10 in]
      }
      frame "Initialize" {
        # "Initialize - Get configuration settings, then message the UI to initialize, and broadcast the settings to the other message loops."
        n146 = property class="VI" props=["FP.State"]() -> (reference out=w396:refnum<vi>)  [unwired: 2 in, 2 out]
        n147 = call-poly "Enqueue Message.vi"("error in (no error)"=w397, "Message"="Init UI Refs", "Message Queue"=w402) -> ("error out"=w400:errorcluster, "dup Message Queue"=w401:refnum<queue>)  [unwired: 7 in]
        n148 = call "Make Child and Move.vi"("Process Name"=w393, "Name of Parent Panel"=w394, "New Center Coords"=w395, "VI in"=w396) -> ()  [unwired: 8 in]
        n149 = call-poly "Enqueue Message.vi"("error in (no error)"=w400, "Message"="Broadcast Settings", "Message Queue"=w401) -> ("error out"=w408:errorcluster, "dup Message Queue"=w407:refnum<queue>)  [unwired: 7 in]
        n150 = call-poly "Enqueue Message.vi"("error in (no error)"=w408, "Message Data"="Ready..." ("Ready..."), "Message"="Update Status", "Message Queue"=w407) -> ("error out"=w389:errorcluster)  [unwired: 6 in, 1 out]
        n151 = Unbundle By Name(w388) -> ("TCU Module Config.Process Name"=w392:string)
        n152 = Concatenate Strings(w392, " Initialize" ("text")) -> (w391:string)
        n153 = call "Write to Log File.vi"("error in"=w389, "text"=w391) -> ()  [unwired: 9 in, 1 out]
      }
      frame "Launch Settings Dialog" {
        # "Launch the Settings Dialog when the user clicks the 'Settings' button."
        n154 = local read "TCU On?"() -> (w411:bool)
        n155 = in-place {
          in-place-border: w411 -> [w426]
          # "Keep track of the # of times the window is opened"
          n156 = in-place-cluster #3(w410) -> ("TCU Module Config.Load Count"=w428:i32)  [unwired: 1 out]
          n157 = Increment(x=w428) -> (x+1=w427:i32)
          n158 = in-place-cluster #3("TCU Module Config.Load Count"=w427, "TCU On?"=w426) -> (w409:T9)
        }
        n159 = call "TCU Settings Dialog.vi"("error in (no error)"=w420, "Message Queues"=w417, "TCU Module State Cluster In"=w409) -> ("error out"=w419:errorcluster, "UI Refresh Needed?"=w418:bool, "TCU Module Config Out"=w421:T2)  [unwired: 5 in, 1 out]
        n160 = case shown="True" w418 {
          tunnel: w419 -> [w431 w437]
          tunnel: [w429 w437] -> w413
          tunnel: w423 -> [_ _]
          tunnel: w422 -> [w430 _]
          frame False {
            n161 = disable-structure shown="Enabled" {
              disable-tunnel: w431 -> [w435 w436]
              disable-tunnel: w430 -> [w434 _]
              disable-tunnel: [w432 w436] -> w429
              frame Disabled {
                n162 = call-poly "Enqueue Message.vi"("error in (no error)"=w435, "Message"="Broadcast Settings", "Message Queue"=w434) -> ("error out"=w432:errorcluster)  [unwired: 7 in, 1 out]
              }
              frame Enabled {
              }
            }
          }
          frame True {
          }
        }
        n163 = Bundle By Name(cluster=w410, "TCU Module Config"=w421) -> (w412:T9)
        n164 = Unbundle By Name(w412) -> ("TCU Module Config.Process Name"=w416:string)
        n165 = Concatenate Strings(w416, " Settings Dialog Launched" ("text")) -> (w415:string)
        n166 = call "Write to Log File.vi"("error in"=w413, "text"=w415) -> ()  [unwired: 9 in, 1 out]
      }
      frame "Logging Stopped" {
        # "Logic for determining what action to take when the logging has stopped."
        n167 = case shown="\"Waiting for Exit (Acq Stopped)\"" w446 {
          selector: w446 -> [w449 _ _ _ _]
          tunnel: [w449 UI_State."Waiting for Exit (Log Stopped)" ("UI State") UI_State."Waiting for Stop (Log Stopped)" ("UI State") UI_State."Idle" ("UI State") UI_State."Idle" ("UI State")] -> w445
          tunnel: w444 -> [w448 w450 w452 w458 w464]
          tunnel: [w448 w450 w452 w457 w463] -> w439
          tunnel: w443 -> [_ _ _ w456 w462]
          frame Default {
          }
          frame "Waiting for Exit", "Waiting for Exit (Log Stopped)" {
          }
          frame "Waiting for Stop", "Waiting for Stop (Log Stopped)" {
          }
          frame "Waiting for Exit (Acq Stopped)" {
            # "If we are waiting to exit, and the acquisition has already stopped, then the \"Logging Stopped\" message indicates that it is time to exit."
            n168 = call-poly "Enqueue Message.vi"("Priority Message? (F)"=TRUE, "error in (no error)"=w458, "Message"="Exit", "Message Queue"=w456) -> ("error out"=w457:errorcluster)  [unwired: 6 in, 1 out]
          }
          frame "Waiting for Stop (Acq Stopped)" {
            # "If we are waiting to stop, and the acquisition has already stopped, then the \"Logging Stopped\" message indicates that it is time to stop."
            n169 = call-poly "Enqueue Message.vi"("error in (no error)"=w464, "Message Data"="Ready..." ("Message"), "Message"="Update Status", "Message Queue"=w462) -> ("error out"=w463:errorcluster)  [unwired: 6 in, 1 out]
          }
        }
        n170 = Unbundle By Name(w438) -> ("TCU Module Config.Process Name"=w442:string)
        n171 = Concatenate Strings(w442, " Logging Stopped" ("text")) -> (w441:string)
        n172 = call "Write to Log File.vi"("error in"=w439, "text"=w441) -> ()  [unwired: 9 in, 1 out]
      }
      frame "Send to Sequence" {
        n173 = Variant To Data(error in=w469, type=refnum<queue> refnum ("Message Queue"), Variant=w466) -> (data=w467:refnum<queue>, error out=w468:errorcluster)
        n174 = local read "Temp Display"() -> (w474:dbl)
        n175 = call-poly "Enqueue Message.vi"("error in (no error)"=w468, "Message Data"=w474, "Message"="Sent to Sequence", "Message Queue"=w467) -> ("error out"=w473:errorcluster)  [unwired: 6 in, 1 out]
      }
      frame "Start" {
        # "Clear chart"
        # "Message Acquisition and Logging loops to start"
        # "Enable: Stop\nDisable: Start, Exit, Settings"
        # "Start - Enable/Disable buttons appropriately for an acquisition that has started, and update status display."
        n176 = Unbundle By Name(w484) -> ("Trigger Ref"=w495:refnum<vi>, "Stop Ref"=w496:refnum<vi>, "Start Ref"=w499:refnum<vi>, "Exit Ref"=w498:refnum<vi>, "Settings Ref"=w497:refnum<vi>, "Data Ref"=w486:refnum<vi>)
        n177 = property class="WFChart (strict)"(reference=w486, "History Data"=waveform(dbl)[][] []) -> ()  [unwired: 1 in, 2 out]
        n178 = Build Array(w499, w498, w497) -> (w502:refnum<vi>[])
        n179 = Build Array(w495, w496) -> (w501:refnum<vi>[])
        n180 = call-poly "Enqueue Message.vi"("error in (no error)"=w487, "Message"="Broadcast settings", "Message Queue"=w489) -> ("error out"=w490:errorcluster, "dup Message Queue"=w488:refnum<queue>)  [unwired: 7 in]
        n181 = call "Set Enable State on Multiple Controls.vi"("Enable?"=TRUE, "Controls"=w501) -> ()  [unwired: 10 in]
        n182 = call "Set Enable State on Multiple Controls.vi"("Enable?"=FALSE, "Controls"=w502) -> ()  [unwired: 10 in]
        n183 = call-poly "Enqueue Message.vi"("error in (no error)"=w490, "Message"="Start Loops", "Message Queue"=w488) -> ("error out"=w491:errorcluster)  [unwired: 7 in, 1 out]
        n184 = Merge Errors(w491) -> (w478:errorcluster)
        n185 = Bundle By Name(cluster=w483, "State"=State_Enum."Measuring") -> (w477:T9)
        n186 = Unbundle By Name(w477) -> ("TCU Module Config.Process Name"=w481:string)
        n187 = Concatenate Strings(w481, " Start" ("text")) -> (w480:string)
        n188 = call "Write to Log File.vi"("error in"=w478, "text"=w480) -> ()  [unwired: 9 in, 1 out]
      }
      frame "Sequence Start" {
        # "Start the sequence if it is not already running"
        # "Clear chart"
        # "Message Acquisition and Logging loops to start"
        # "Enable: Stop\nDisable: Start, Exit, Settings"
        # "Start - Enable/Disable buttons appropriately for an acquisition that has started, and update status display."
        n189 = Unbundle By Name(w516) -> ("Trigger Ref"=w523:refnum<vi>, "Stop Ref"=w524:refnum<vi>, "Start Ref"=w527:refnum<vi>, "Exit Ref"=w526:refnum<vi>, "Settings Ref"=w525:refnum<vi>, "Data Ref"=w518:refnum<vi>)
        n190 = property class="WFChart (strict)"(reference=w518, "History Data"=waveform(dbl)[][] []) -> ()  [unwired: 1 in, 2 out]
        n191 = Build Array(w527, w526, w525) -> (w530:refnum<vi>[])
        n192 = Build Array(w523, w524) -> (w529:refnum<vi>[])
        n193 = call-poly "Enqueue Message.vi"("error in (no error)"=w519, "Message"="Broadcast settings", "Message Queue"=w520) -> ("error out"=w512:errorcluster, "dup Message Queue"=w513:refnum<queue>)  [unwired: 7 in]
        n194 = call "Set Enable State on Multiple Controls.vi"("Enable?"=TRUE, "Controls"=w529) -> ()  [unwired: 10 in]
        n195 = call "Set Enable State on Multiple Controls.vi"("Enable?"=FALSE, "Controls"=w530) -> ()  [unwired: 10 in]
        n196 = case shown="False" w510 {
          selector: w510 -> [_ w537]
          tunnel: [TRUE w537] -> w509
          tunnel: w512 -> [w535 w538]
          tunnel: w513 -> [w533 _]
          tunnel: [w532 w538] -> w511
          frame False {
            n197 = call-poly "Enqueue Message.vi"("error in (no error)"=w535, "Message"="Start Loops", "Message Queue"=w533) -> ("error out"=w532:errorcluster)  [unwired: 7 in, 1 out]
          }
          frame True {
          }
        }
        n198 = Merge Errors(w511) -> (w505:errorcluster)
        n199 = Bundle By Name(cluster=w515, "State"=State_Enum."Measuring") -> (w504:T9)
        n200 = Unbundle By Name(w504) -> ("TCU Module Config.Process Name"=w508:string)
        n201 = Concatenate Strings(w508, " Sequence Start" ("text")) -> (w507:string)
        n202 = call "Write to Log File.vi"("error in"=w505, "text"=w507) -> ()  [unwired: 9 in, 1 out]
      }
      frame "Start Loops" {
        # "We don't have multiple Process Names per module, but i am leaving it for now."
        # "Message Acquisition and Logging loops to start"
        # "Start - Enable/Disable buttons appropriately for an acquisition that has started, and update status display."
        n203 = Unbundle By Name(w540) -> ("TCU Module Config.Process Name"=w541:string)
        n204 = Build Array(w544) -> (w542:refnum<queue>[])
        n205 = for {
          tunnel: w539 -> [w551]
          tunnel: [w550] -> w543 mode=indexing
          tunnel: w542 -> [w549] mode=indexing
          tunnel: w541 -> [w548]
          n206 = call-poly "Enqueue Message.vi"("error in (no error)"=w551, "Message Data"=w548, "Message"="Start", "Message Queue"=w549) -> ("error out"=w550:errorcluster)  [unwired: 6 in, 1 out]
        }
        n207 = property class="VI"("Front Panel.Title"=w541) -> ()  [unwired: 2 in, 2 out]
        n208 = Merge Errors(w539, w543) -> (w547:errorcluster)
      }
      frame "Start Log" {
        # "Message Acquisition and Logging loops to start"
        # "Start - Enable/Disable buttons appropriately for an acquisition that has started, and update status display."
        n209 = Unbundle By Name(w554) -> ("TCU Module Config.Process Name"=w559:string)
        n210 = Build Array(w562) -> (w560:refnum<queue>[])
        n211 = for {
          tunnel: w553 -> [w568]
          tunnel: [w567] -> w561 mode=indexing
          tunnel: w560 -> [w566] mode=indexing
          tunnel: w559 -> [w565]
          n212 = call-poly "Enqueue Message.vi"("error in (no error)"=w568, "Message Data"=w565, "Message"="Start Log", "Message Queue"=w566) -> ("error out"=w567:errorcluster)  [unwired: 6 in, 1 out]
        }
        n213 = property class="VI"("Front Panel.Title"=w559) -> ()  [unwired: 2 in, 2 out]
        n214 = Merge Errors(w553, w561) -> (w555:errorcluster)
        n215 = Unbundle By Name(w554) -> ("TCU Module Config.Process Name"=w558:string)
        n216 = Concatenate Strings(w558, " Start Log" ("text")) -> (w557:string)
        n217 = call "Write to Log File.vi"("error in"=w555, "text"=w557) -> ()  [unwired: 9 in, 1 out]
      }
      frame "Stop" {
        # "Pause the TCU on Stop"
        # "Enable: Start, Exit, Settings\nDisable: Stop"
        # "Stop - Enable/Disable buttons appropriately for an acquisition that has stopped, and update status display."
        n218 = Unbundle By Name(w597) -> ("Trigger Ref"=w588:refnum<vi>, "Stop Ref"=w589:refnum<vi>, "Start Ref"=w592:refnum<vi>, "Exit Ref"=w591:refnum<vi>, "Settings Ref"=w590:refnum<vi>)
        n219 = call-poly "Enqueue Message.vi"("error in (no error)"=w571, "Message"="Broadcast settings", "Message Queue"=w573) -> ("error out"=w570:errorcluster, "dup Message Queue"=w572:refnum<queue>)  [unwired: 7 in]
        n220 = Build Array(w592, w591, w590) -> (w595:refnum<vi>[])
        n221 = Build Array(w588, w589) -> (w594:refnum<vi>[])
        n222 = call-poly "Enqueue Message.vi"("error in (no error)"=w570, "Message Data"="Ready..." ("Ready..."), "Message"="Update Status", "Message Queue"=w572) -> ("error out"=w584:errorcluster)  [unwired: 6 in, 1 out]
        n223 = call "Set Enable State on Multiple Controls.vi"("Enable?"=FALSE, "Controls"=w594) -> ()  [unwired: 10 in]
        n224 = call "Set Enable State on Multiple Controls.vi"("Enable?"=TRUE, "Controls"=w595) -> ()  [unwired: 10 in]
        n225 = call-poly "Enqueue Message.vi"("error in (no error)"=w584, "Message"="Pause", "Message Queue"=w585) -> ("error out"=w582:errorcluster)  [unwired: 7 in, 1 out]
        n226 = case shown="\"Waiting for Exit\"" w586 {
          selector: w586 -> [_ w601]
          tunnel: [UI_State."Waiting for Stop" ("UI State") w601] -> w587
          frame Default {
          }
          frame "Waiting for Exit" {
          }
        }
        n227 = Merge Errors(w582) -> (w576:errorcluster)
        n228 = Bundle By Name(cluster=w581, "State"=State_Enum."Paused") -> (w575:T9)
        n229 = Unbundle By Name(w575) -> ("TCU Module Config.Process Name"=w579:string)
        n230 = Concatenate Strings(w579, " Stop" ("text")) -> (w578:string)
        n231 = call "Write to Log File.vi"("error in"=w576, "text"=w578) -> ()  [unwired: 9 in, 1 out]
      }
      frame "Update Status" {
        # "Update Display - Convert the message data to a string to display in the Status indicator."
        n232 = Variant To Data(error in=w612, type="", Variant=w611) -> (data=w605:string, error out=w609:errorcluster)
        "Status" <- w605
        n233 = Unbundle By Name(w608) -> ("Trigger Ref"=w604:refnum<vi>, "Stop Ref"=w607:refnum<vi>)
        n234 = property class="Bool"(reference=w607) -> ("DisabledEnum"=w606:T17)  [unwired: 1 in, 2 out]
        n235 = case shown="\"Enabled\"" w606 {
          tunnel: w605 -> [w616 _]
          tunnel: w604 -> [w617 _]
          frame "Enabled" {
            # "Disable the Force Trigger only while we are logging."
            n236 = Build Array(w617) -> (w618:refnum<vi>[])
            n237 = Not Equal?(x="Logging" ("Logging"), y=w616) -> (x != y?=w614:bool)
            n238 = call "Set Enable State on Multiple Controls.vi"("Enable?"=w614, "Controls"=w618) -> ()  [unwired: 10 in]
          }
          frame "Disabled", Default {
          }
        }
        n239 = Merge Errors(w609) -> (w613:errorcluster)
      }
      frame Default {
        # "'Default' case only runs if there is a message that isn't defined in any of the other cases.  Output a programming error."
        n240 = Concatenate Strings("The invalid message string " ("string"), w620, " was received in TCU Main." ("string")) -> (w621:string)
        n241 = Bundle By Name(cluster=errorcluster {"status"=TRUE, "code"=1, "source"=""} ("error constant"), "source"=w621) -> (w619:errorcluster)
        n242 = Unbundle By Name(w625) -> ("TCU Module Config.Process Name"=w628:string)
        n243 = Concatenate Strings(w628, " Incorrect Message Recieved: " ("text"), w620) -> (w627:string)
        n244 = call "Write to Log File.vi"("error in"=w619, "text"=w627) -> ()  [unwired: 9 in, 1 out]
      }
    }
    n245 = call "Error Handler - Message Handling Loop.vi"("error in (no error)"=w110, "Message Queue"=w108) -> ("dup error in"=w109:errorcluster, "dup Message Queue"=w94:refnum<queue>)  [unwired: 8 in]
  }
  n246 = call "Main Loop.vi"("error in (no error)"=w9, "Chart Notifier"=w23, "Message Queues"=w10) -> ("error out"=w24:errorcluster)  [unwired: 8 in]
  n247 = Release Queue(queue=w3) -> ()  [unwired: 2 in, 3 out]
  n248 = Release Queue(queue=w2) -> ()  [unwired: 2 in, 3 out]
  n249 = Close Reference(reference=w22) -> ()  [unwired: 1 in, 1 out]
  n250 = Unregister For Events(event registration refnum=w32, error in=w37) -> (error out=w33:errorcluster)
  n251 = Merge Errors(w33, w38, w9, w24) -> (w36:errorcluster)
  n252 = Release Queue(queue=w1) -> ()  [unwired: 2 in, 3 out]
  n253 = call "Destroy User Event - Stop.vi"("error in (no error)"=w36, "User Event - Stop"=w34) -> ()  [unwired: 9 in, 1 out]
